vi "Open Camera Stream.vi"(0 "video in":refnum<class "MSC Video.lvclass">, 1 "CamID":i32, 2 "Camera API":T1 items=["Auto", "MIL proprietary drivers", "VFW platform native, V4L, V4L2", "Fireware, Firewire, IEEE 1394, DC 1394, CMU 1394", "Stereo TYZX proprietary drivers", "Quicktime", "Unicap", "DirectShow", "PvAPI, Prosilica GigE SDK", "OpenNI (Kinect)", "Android", "XIMEA Camera", "AVFoundation framework"], 5 "error in (no error)":errorcluster) -> (14 "video out":refnum<class "MSC Video.lvclass">, 19 "error out":errorcluster)   [LabVIEW 2014, in "MSC Video.lvclass"]
doc: "Starts a camera stream with the selected camera with CamID.\n\nThe camera API is selected automatically. It is also possible to select a specific one with Camera API."
uses:
  MSC Video.lvclass
  controls/Camera API.ctl
  MSC Video.lvclass/MSC Video.ctl
  Dependencies/x86/MSC I Process32.dll
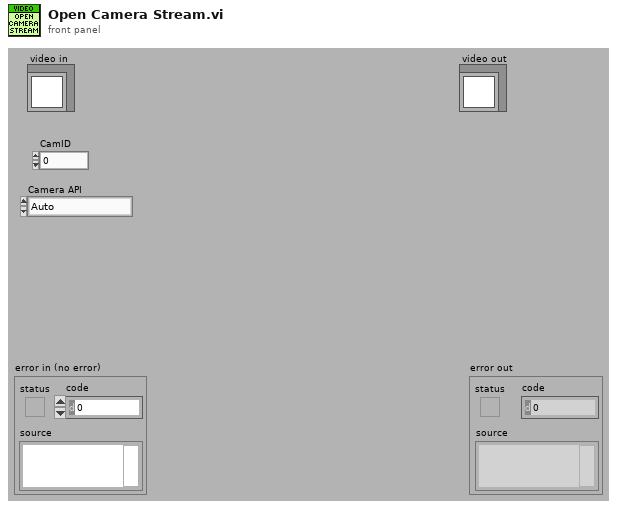
[diagram p1: front panel]
types:
  T1 = typedef "MSC Video.lvclass/Camera API.ctl" = u16
  T2 = typedef "MSC Video.lvclass/Video.ctl" = cluster{"Pointer":u64, "CamID":i32, "File Path":path, "Network Address":string, "opened":bool}
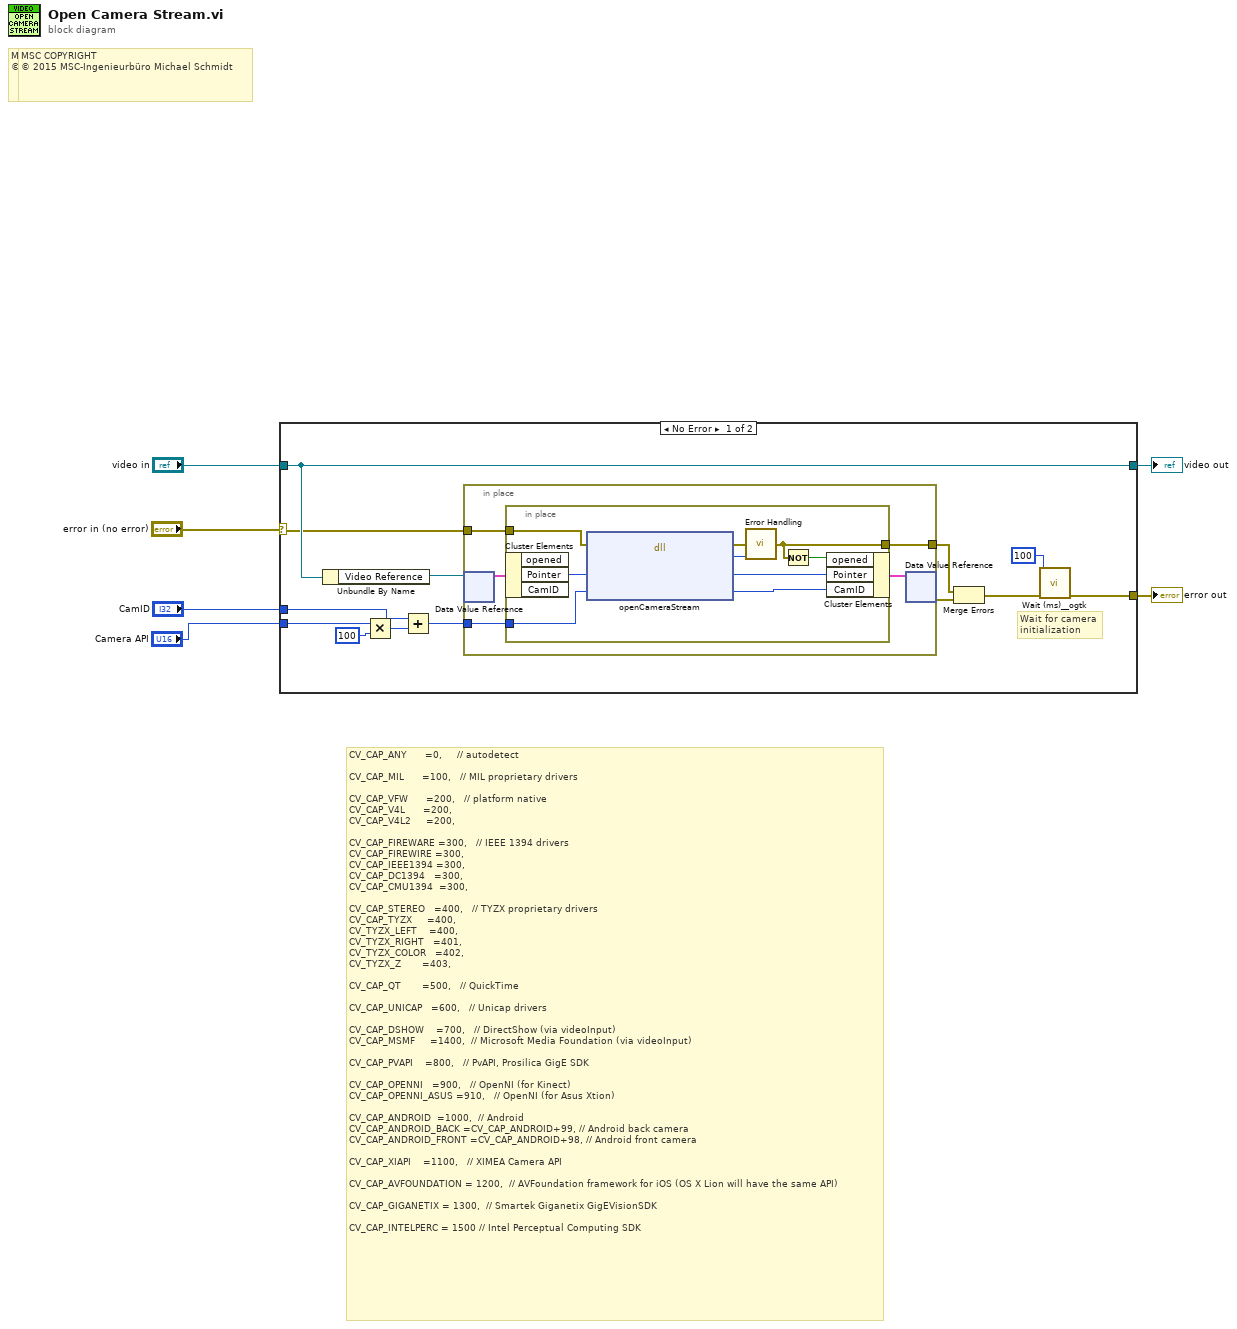
[diagram p0: block diagram]
diagram:
  # "MSC COPYRIGHT\n© 2016 MSC-Ingenieurbüro Michael Schmidt"
  # "MSC COPYRIGHT\n© 2016 MSC-Ingenieurbüro Michael Schmidt"
  # "MSC COPYRIGHT\n© 2015 MSC-Ingenieurbüro Michael Schmidt"
  # "CV_CAP_ANY      =0,     // autodetect\n\nCV_CAP_MIL      =100,   // MIL proprietary drivers\n\nCV_CAP_VFW      =200,   // platform native\nCV_CAP_V4L      =200,\nCV_CAP_V4L2     =200,\n\nCV_CAP_FIREWARE =300,   // IEEE 1394 drivers\nCV_CAP_FIREWIRE =300,\nCV_CAP_IEEE1394 =300,\nCV_CAP_DC1394   =300,\nCV_CAP_CMU1394  =300,\n\nCV_CAP_STEREO   =400,   // TYZX proprietary drivers\nCV_CAP_TYZX     =400,\nCV_TYZX_LEFT    =400,\nCV_TYZX_RIGHT   =401,\nCV_TYZX_COLOR   =402,\nCV_TYZX_Z       =403,\n\nCV_CAP_QT       =500,   // QuickTime\n\nCV_CAP_UNICAP   =600,   // Unicap drivers\n\nCV_CAP_DSHOW    =700,   // DirectShow (via videoInput)\nCV_CAP_MSMF     =1400,  // Microsoft Media Foundation (via videoInput)\n\nCV_CAP_PVAPI    =800,   // PvAPI, Prosilica GigE SDK\n\nCV_CAP_OPENNI   =900,   // OpenNI (for Kinect)\nCV_CAP_OPENNI_ASUS =910,   // OpenNI (for Asus Xtion)\n\nCV_CAP_ANDROID  =1000,  // Android\nCV_CAP_ANDROID_BACK =CV_CAP_ANDROID+99, // Android back camera\nCV_CAP_ANDROID_FRONT =CV_CAP_ANDROID+98, // Android front camera\n\nCV_CAP_XIAPI    =1100,   // XIMEA Camera API\n\nCV_CAP_AVFOUNDATION = 1200,  // AVFoundation framework for iOS (OS X Lion will have the same API)\n\nCV_CAP_GIGANETIX = 1300,  // Smartek Giganetix GigEVisionSDK\n\nCV_CAP_INTELPERC = 1500 // Intel Perceptual Computing SDK"
  n1 = case shown="No Error" "error in (no error)" {
    selector: "error in (no error)" -> [w14 w35]
    tunnel: [w11 w35] -> w5
    tunnel: "video in" -> [w15 w34]
    tunnel: [w15 w34] -> w3
    tunnel: "CamID" -> [w13 _]
    tunnel: "Camera API" -> [w12 _]
    frame No Error {
      # "Wait for camera\ninitialization"
      n2 = Unbundle By Name(w15) -> ("Video Reference"=w16:refnum<data-value>)
      n3 = Multiply(x=w12, y=100) -> (x*y=w7:i32)
      n4 = Add(x=w13, y=w7) -> (x+y=w17:i32)
      n5 = in-place {
        in-place-border: [w22] -> w18
        in-place-border: w17 -> [w21]
        in-place-border: w14 -> [w20]
        n6 = in-place-dvr #1(w16) -> (w23:T2)  [unwired: 1 out]
        n7 = in-place {
          in-place-border: [w28] -> w22
          in-place-border: w21 -> [w31]
          in-place-border: w20 -> [w25]
          n8 = in-place-cluster #2(w23) -> ("Pointer"=w33:u64)  [unwired: 2 out]
          n9 = dll-call lib="C:/Users/MSC/LabVIEW Projekte/LV 2014/MSC I-Process/user.lib/MSC-I Process/Dependencies/x86/MSC I Process*.dll" fn="openCameraStream"(error in=w25, "pointer"=w33, "camID"=w31) -> (error out=w30:errorcluster, "error"=w29:i32, "pointer"=w26:u64, "camID"=w32:i32)  [unwired: 2 in, 1 out]
          n10 = call "Error Handling.vi"("error in (no error)"=w30, "return type"=w29) -> ("error out"=w28:errorcluster)  [unwired: 12 in, 1 out]
          n11 = Not(x=w28) -> (.not. x?=w27:bool)
          n12 = in-place-cluster #2("opened"=w27, "Pointer"=w26, "CamID"=w32) -> (w24:T2)
        }
        n13 = in-place-dvr #1(w24) -> (w19:errorcluster)  [unwired: 1 out]
      }
      n14 = Merge Errors(w18, w19) -> (w10:errorcluster)
      n15 = call <userlib>:"Wait (ms)__ogtk.vi"("error in (no error)"=w10, "milliseconds to wait"=u32 100) -> ("error out"=w11:errorcluster)  [unwired: 8 in, 1 out]
    }
    frame Error {
    }
  }
  "error out" <- w5
  "video out" <- w3
